vi "Query Output.vi"(8 "error in":errorcluster, 11 "6512 in":refnum<class "6512.lvclass">) -> (0 "error out":errorcluster, 1 "Boolean array":bool[](array[boolean]), 2 "Port Array":u8[](array[numeric]), 3 "6512 out":refnum<class "6512.lvclass">)   [LabVIEW 2019, in "6512.lvlib" / "6512.lvclass"]
uses:
  Library/6512.lvclass
  Library/6512.lvclass/6512.ctl
  <vilib>/DAQmx/read.llb/DAQmx Read (Digital 1D U8 NChan 1Samp).vi
  <vilib>/DAQmx/miscellaneous.llb/DAQmx Fill In Error Info.vi
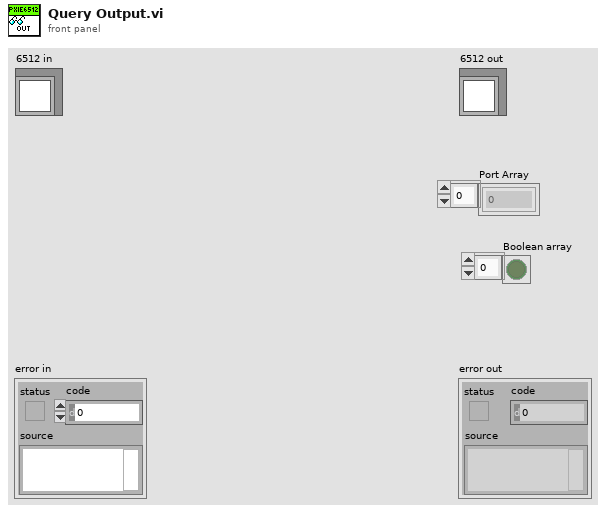
[diagram p1: front panel]
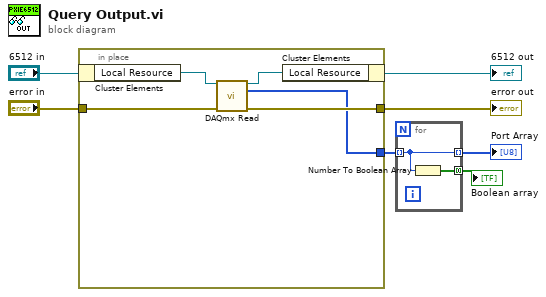
[diagram p0: block diagram]
diagram:
  n1 = in-place {
    in-place-border: "error in" -> [w10]
    in-place-border: [w9] -> w4
    in-place-border: [w8] -> w3
    n2 = in-place-cluster #1("6512 in") -> ("Local Resource"=w12:refnum<k21>)
    n3 = call-poly <vilib>:"DAQmx Read.vi"("task/channels in"=w12, "error in"=w10) -> ("task out"=w11:refnum<k21>, "data"=w8:u8[], "error out"=w9:errorcluster)  [unwired: 11 in]
    n4 = in-place-cluster #1("Local Resource"=w11) -> (→"6512 out":refnum<class "6512.lvclass">)
  }
  "error out" <- w4
  n5 = for {
    tunnel: w3 -> [w14] mode=indexing
    tunnel: [w14] -> w2 mode=indexing
    tunnel: [w13] -> w1 mode=concatenating
    n6 = Number To Boolean Array(number=w14) -> (Boolean array=w13:bool[])
  }
  "Port Array" <- w2
  "Boolean array" <- w1
